vi "test_set_excitation_LS372.vi"() -> ()   [LabVIEW 2018]
uses:
  Instrument_Setup.vi
  Equipment/Lake Shore 372/Lake Shore 372.lvlib
panel:
  out "Numeric":dbl
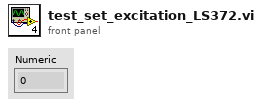
[diagram p1: front panel]
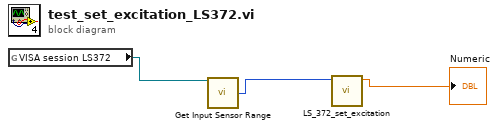
[diagram p0: block diagram]
diagram:
  n1 = global read "Instrument_Setup.vi" "VISA session LS372"() -> (w3:refnum<visa-resource-name>)
  n2 = call "Get Input Sensor Range.vi"("VISA resource name"=w3) -> ("Excitation Range"=w2:u16)  [unwired: 7 in, 7 out]
  n3 = call "LS_372_set_excitation.vi"("LS_Excitation old"=w2) -> ("LS_Excitation new"=→"Numeric":dbl)  [unwired: 5 in, 1 out]
